vi "Calibirattionvi.vi"() -> ()   [LabVIEW 2013]
panel:
  out "Image Out 2":T1(plugin-control)
  out "Image Out":T1(plugin-control)
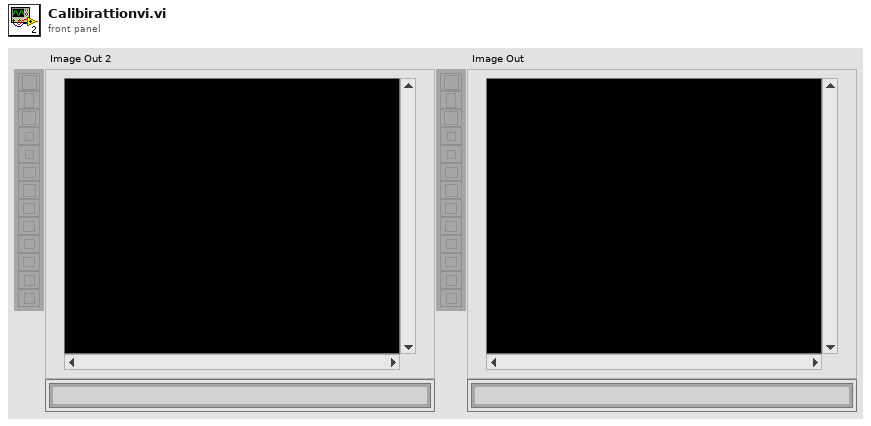
[diagram p1: front panel]
types:
  T1 = typedef "IMAQ Image.ctl" = refnum<image>
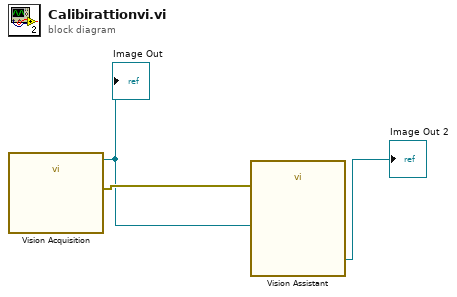
[diagram p0: block diagram]
diagram:
  n1 = call "Vision Acquisition"() -> ("Image Out"=w2:T1, "error out"=w3:errorcluster)  [unwired: 26 in]
  "Image Out" <- w2
  n2 = call "Vision Assistant"("Image In"=w2, "error in"=w3) -> ("Image Out"=→"Image Out 2":T1)  [unwired: 24 in, 1 out]
